vi "Write IInstrument Base.vi"(8 "error in (no error)":errorcluster, 10 "IInstrument Base":refnum<class "IInstrument.lvclass">, 11 "Virtual Instrument Base in":refnum<class "Virtual Instrument Base.lvclass">) -> (0 "error out":errorcluster, 3 "Virtual Instrument Base out":refnum<class "Virtual Instrument Base.lvclass">)   [LabVIEW 2023, in "HAL GOOP4.lvlib" / "Virtual Instrument Base.lvclass"]
uses:
  Virtual Instrument Base.lvclass
  Virtual Instrument Base.lvclass/Virtual Instrument Base.ctl
  Interfaces/IInstrument/IInstrument.lvclass
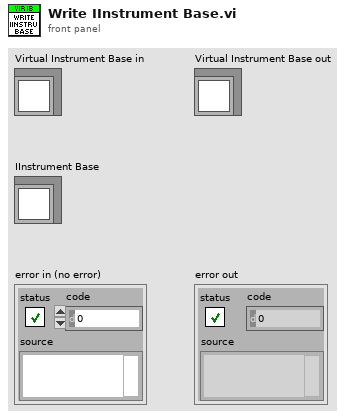
[diagram p1: front panel]
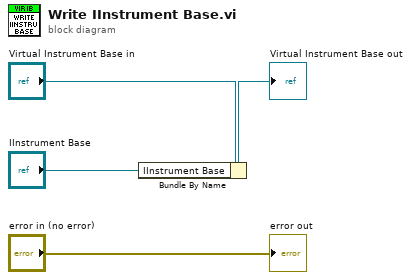
[diagram p0: block diagram]
diagram:
  n1 = Bundle By Name(cluster="Virtual Instrument Base in", "IInstrument Base"="IInstrument Base") -> (→"Virtual Instrument Base out":refnum<class "Virtual Instrument Base.lvclass">)
  "error out" <- "error in (no error)"
